vi "DOM coag demand.vi"(8 "error in (no error)":errorcluster, 10 "averaged data":T1, 11 "Coagulant":T2={"flocculator volume (L)"=100.0, "clarifier volume (L)"=0.0, "dose updates per HRT"=0, "target clarified turbidity (NTU)"=0.3, "Coagulant mode"=enum."manual", "Coag dose [mg/L]"=0.0, "pump mL/rev"=0.0, "clarifier flow [L/s]"=0.5, "min Coag dose [mg/L]"=0.0, "max Coag dose [mg/L]"=0.0, "Steps"=3, "HRT response delay"=1, "kpf"=1.0, "DOM coag demand [mg/L]"=0.0, "min DOM coag demand [mg/L]"=0.0, "max DOM coag demand [mg/L]"=0.0} {"max DOM coag demand [mg/L]" min=0.0 max=20.0 step=0.1; "min DOM coag demand [mg/L]" min=0.0 max=10.0 step=0.1; "DOM coag demand [mg/L]" min=0.0 max=20.0 step=0.1; "HRT response delay" min=1 max=10 step=1; "Steps" min=3 step=1; "clarifier flow [L/s]" min=0.0001 max=1.0 step=0.0001; "target clarified turbidity (NTU)" min=0.1 max=5.0 step=0.01; "dose updates per HRT" min=1 max=100 step=1}) -> (0 "error out":errorcluster, 1 "In Range?":bool, 2 "averaged data with coag demand":T1, 3 "DOM coag demand":dbl)   [LabVIEW 2019]
uses:
  coag.ctl
  model type.ctl
  data cluster.ctl
  Sensor buffer command.ctl
panel:
  # "ramp controls"
  # "min"
  # "max"
  # "min"
  # "max"
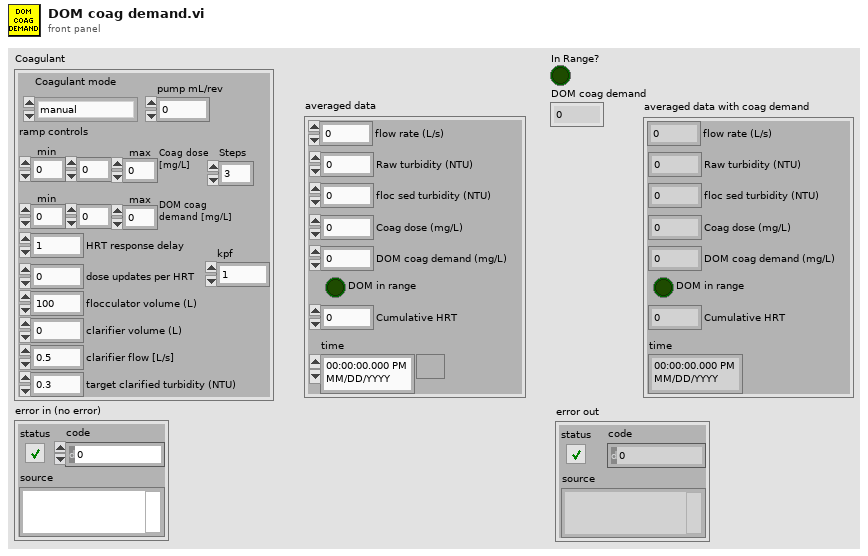
[diagram p1: front panel]
types:
  T1 = typedef "data cluster.ctl" = cluster{"floc sed turbidity (NTU)":dbl, "Raw turbidity (NTU)":dbl, "flow rate (L/s)":dbl, "time":timestamp, "Cumulative HRT":dbl, "Coag dose (mg/L)":dbl, "DOM coag demand (mg/L)":dbl, "DOM in range":bool}
  T2 = typedef "coag.ctl" = cluster{"flocculator volume (L)":dbl, "clarifier volume (L)":dbl, "dose updates per HRT":u16, "target clarified turbidity (NTU)":dbl, "Coagulant mode":T3, "Coag dose [mg/L]":dbl, "pump mL/rev":dbl, "clarifier flow [L/s]":dbl, "min Coag dose [mg/L]":dbl, "max Coag dose [mg/L]":dbl, "Steps":u16, "HRT response delay":u32, "kpf":dbl, "DOM coag demand [mg/L]":dbl, "min DOM coag demand [mg/L]":dbl, "max DOM coag demand [mg/L]":dbl}
  T3 = typedef "model type.ctl" = enum16{"manual", "ramp", "simple corrector"}
  T4 = typedef "Sensor buffer command.ctl" = enum16{"set buffer size", "write", "refill buffer", "read recent", "read all", "read at delta HRT", "clear"}
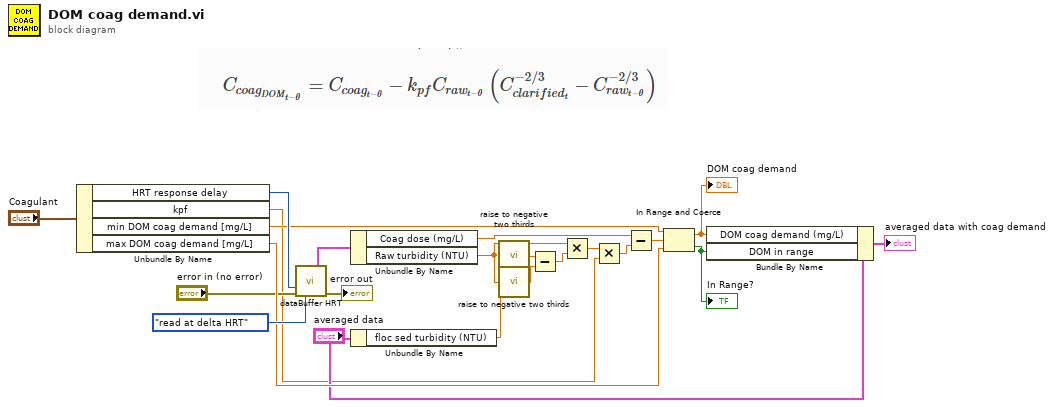
[diagram p0: block diagram]
diagram:
  n1 = Unbundle By Name("Coagulant") -> ("HRT response delay"=w21:u32, "kpf"=w2:dbl, "min DOM coag demand [mg/L]"=w17:dbl, "max DOM coag demand [mg/L]"=w16:dbl)
  n2 = call "dataBuffer HRT.vi"("delta HRT"=w21, "error in (no error)"="error in (no error)", "command"=Sensor_buffer_command."read at delta HRT") -> ("recent at deltaHRT"=w20:T1, "error out"=→"error out":errorcluster)  [unwired: 7 in, 4 out]
  n3 = Unbundle By Name(w20) -> ("Coag dose (mg/L)"=w9:dbl, "Raw turbidity (NTU)"=w5:dbl)
  n4 = Unbundle By Name("averaged data") -> ("floc sed turbidity (NTU)"=w8:dbl)
  n5 = call "raise to negative two thirds.vi"("Numeric in"=w8) -> ("Numeric out"=w7:dbl)  [unwired: 4 in]
  n6 = call "raise to negative two thirds.vi"("Numeric in"=w5) -> ("Numeric out"=w6:dbl)  [unwired: 4 in]
  n7 = Subtract(x=w7, y=w6) -> (x-y=w4:dbl)
  n8 = Multiply(x=w5, y=w4) -> (x*y=w3:dbl)
  n9 = Multiply(x=w3, y=w2) -> (x*y=w1:dbl)
  n10 = Subtract(x=w9, y=w1) -> (x-y=w18:dbl)
  n11 = In Range and Coerce(upper limit=w17, x=w18, lower limit=w16) -> (coerced(x)=w12:dbl, In Range?=w11:bool)
  "In Range?" <- w11
  "DOM coag demand" <- w12
  n12 = Bundle By Name(cluster="averaged data", "DOM coag demand (mg/L)"=w12, "DOM in range"=w11) -> (→"averaged data with coag demand":T1)
